vi "GetParentsChildsGen.vi"(8 "ErrorIn(No Error)":errorcluster caption="entrée d'erreur (pas d'erreur)", 10 "ParentTag":string, 11 "TreeRef":refnum<vi>) -> (0 "sortie d'erreur":errorcluster, 2 "Childs":string[](array[string]), 3 "TreeRef Out":refnum<vi>)   [LabVIEW 2012]
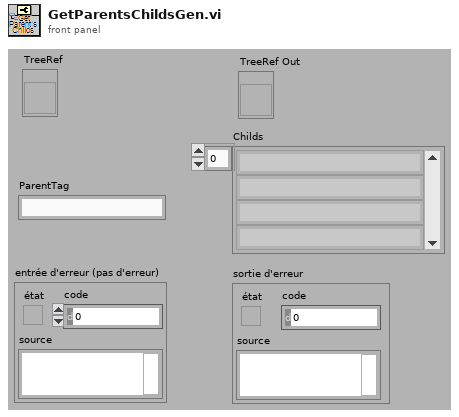
[diagram p1: front panel]
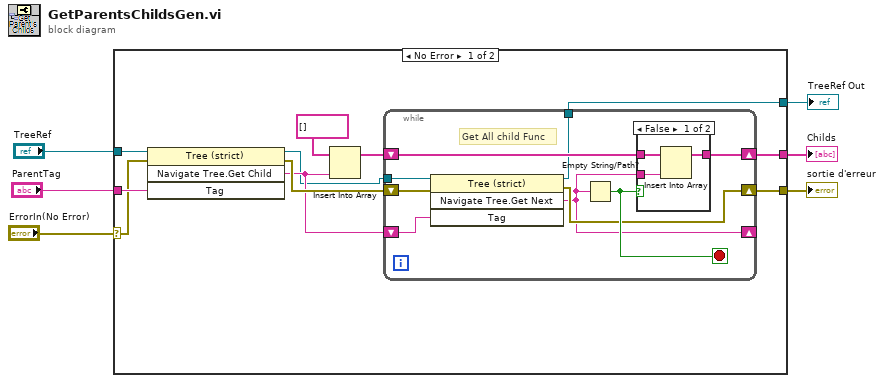
[diagram p0: block diagram]
diagram:
  n1 = case shown="No Error" "ErrorIn(No Error)" {
    selector: "ErrorIn(No Error)" -> [w11 w32]
    tunnel: "ParentTag" -> [w14 _]
    tunnel: [w13 _] -> w5
    tunnel: "TreeRef" -> [w12 w31]
    tunnel: [w10 w32] -> w2
    tunnel: [w9 w31] -> w1
    frame No Error {
      n2 = invoke on="Nœud de méthode" class="Tree (strict)" method="Navigate Tree.Get Child"(reference=w12, error in=w11, "Tag"=w14) -> (reference out=w7:refnum<vi>, error out=w17:errorcluster, "Navigate Tree:Get Child"=w8:string)  [unwired: 1 in, 1 out]
      n3 = Insert Into Array(array=string[] [] ("tableau"), new element=w8) -> (w15:string[])  [unwired: 1 in]
      n4 = while {
        shift-right: [w26] -> w13
        shift-left: w15 -> [w24]
        shift-right: [w22] -> w10
        shift-left: w17 -> [w23]
        tunnel: w7 -> [w21]
        tunnel: [w20] -> w9
        shift-right: [w19] -> _
        shift-left: w8 -> [w18]
        stop <- w25 stop-if-true
        # "Get All child Func"
        n5 = invoke on="Nœud de méthode" class="Tree (strict)" method="Navigate Tree.Get Next"(reference=w21, error in=w23, "Tag"=w18) -> (reference out=w20:refnum<vi>, error out=w22:errorcluster, "Navigate Tree:Get Next Item"=w19:string)  [unwired: 1 in, 1 out]
        n6 = Empty String/Path?(string/path=w19) -> (empty?=w25:bool)
        n7 = case shown="False" w25 {
          tunnel: [w29 w30] -> w26
          tunnel: w19 -> [w28 _]
          tunnel: w24 -> [w27 w30]
          frame False {
            n8 = Insert Into Array(array=w27, new element=w28) -> (w29:string[])  [unwired: 1 in]
          }
          frame True {
          }
        }
      }
    }
    frame Error {
    }
  }
  "Childs" <- w5
  "sortie d'erreur" <- w2
  "TreeRef Out" <- w1
